vi "Is Property Node.vi"(11 "Affected Items":T1) -> (3 "Property Node?":bool)   [LabVIEW 2023]
doc: "Determine if selected BD object is a property node"
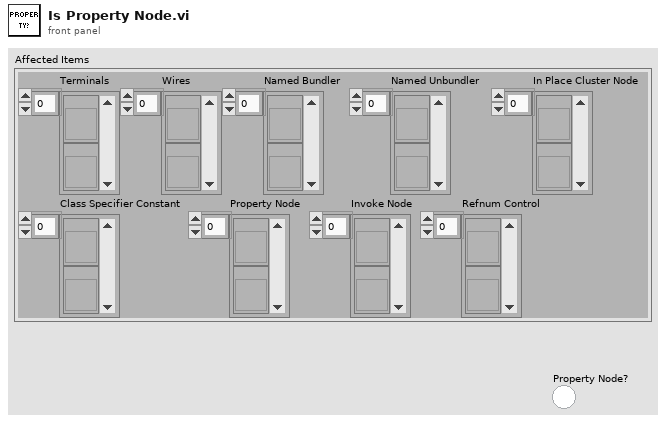
[diagram p1: front panel]
types:
  T1 = cluster{"Terminals":refnum<vi>[], "Wires":refnum<vi>[], "Named Bundler":refnum<vi>[], "Named Unbundler":refnum<vi>[], "In Place Cluster Node":refnum<vi>[], "Class Specifier Constant":refnum<vi>[], "Property Node":refnum<vi>[], "Invoke Node":refnum<vi>[], "Refnum Control":refnum<vi>[]}
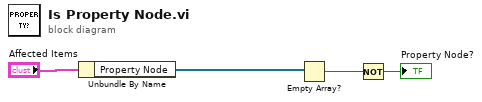
[diagram p0: block diagram]
diagram:
  n1 = Unbundle By Name("Affected Items") -> ("Property Node"=w3:refnum<vi>[])
  n2 = Empty Array?(array=w3) -> (empty?=w2:bool)
  n3 = Not(x=w2) -> (.not. x?=→"Property Node?":bool)
